vi "连接机柜.vi"(8 "error in (no error)":errorcluster) -> (0 "error out":errorcluster)   [LabVIEW 2015]
uses:
  Global/SeverGlobal.vi
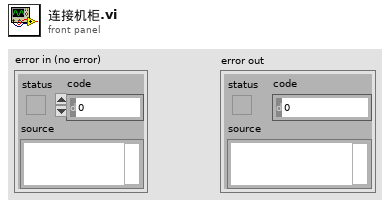
[diagram p1: front panel]
types:
  T1 = cluster{"IP_A":string, "PORT_A":i32, "IP_B":string, "PORT_B":i32, "IP_CLK":string, "PORT_CLK":i32, "IP_SWITCH":string, "PORT_SWITCH":i32}
  T2 = enum16{"Standard", "Buffered", "CRLF", "Immediate"}
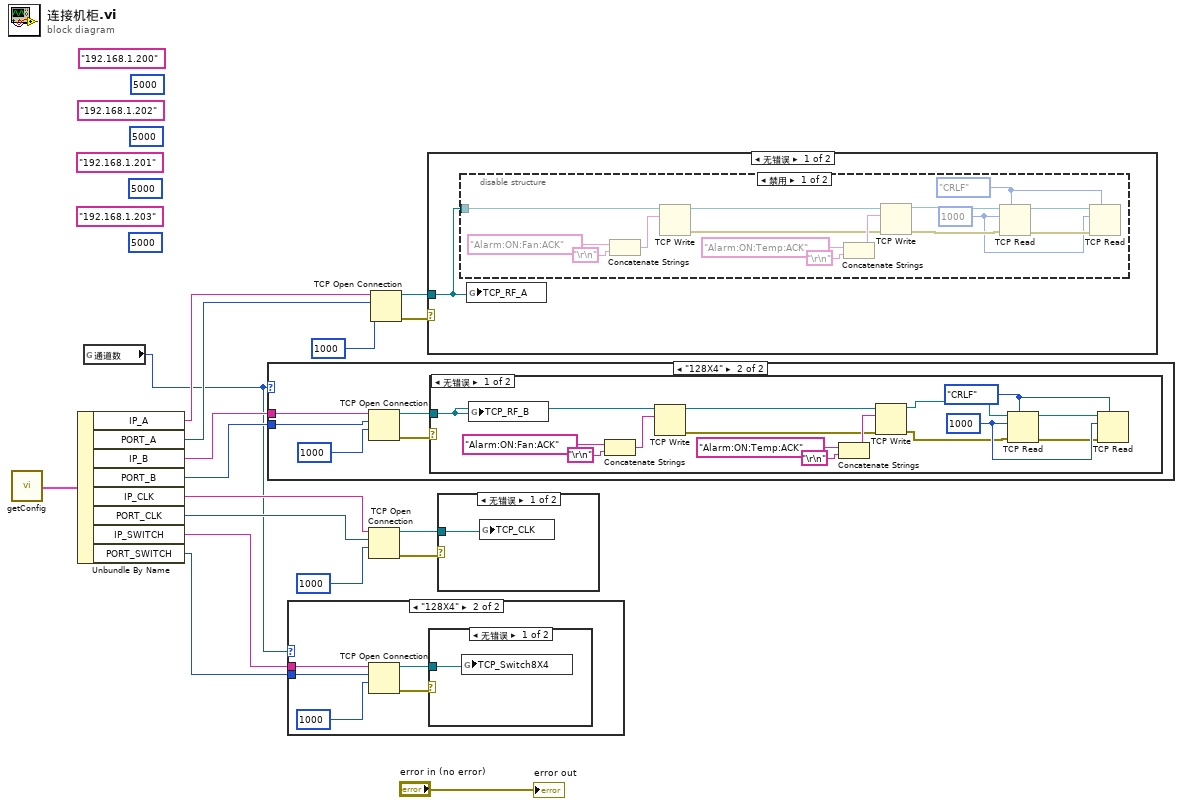
[diagram p0: block diagram]
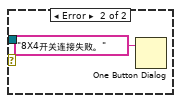
[diagram p3: hidden frame]
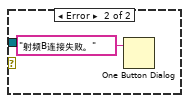
[diagram p5: hidden frame]
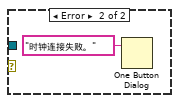
[diagram p6: hidden frame]
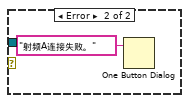
[diagram p8: hidden frame]
diagram:
  (unwired) u16 5000 ("PORT(RF)")
  (unwired) "192.168.1.203" ("IP(RF2)")
  (unwired) u16 5000 ("PORT(RF)")
  (unwired) "192.168.1.201" ("IP(RF2)")
  (unwired) u16 5000 ("PORT(RF)")
  (unwired) "192.168.1.202" ("IP(RF2)")
  (unwired) u16 5000 ("PORT(RF)")
  (unwired) "192.168.1.200" ("IP(RF2)")
  n1 = call "getConfig.vi"() -> ("config"=w10:T1)  [unwired: 1 in]
  n2 = Unbundle By Name(w10) -> ("IP_A"=w9:string, "PORT_A"=w8:i32, "IP_B"=w7:string, "PORT_B"=w6:i32, "IP_CLK"=w5:string, "PORT_CLK"=w4:i32, "IP_SWITCH"=w3:string, "PORT_SWITCH"=w2:i32)
  n3 = global read "SeverGlobal.vi" "通道数"() -> (w1:enum16{"64X4", "128X4"})
  n4 = case shown="\"128X4\"" w1 {
    tunnel: w7 -> [_ w19]
    tunnel: w6 -> [_ w18]
    frame "64X4", Default {
    }
    frame "128X4" {
      n5 = TCP Open Connection(address=w19, remote port or service name=w18, timeout ms (60000)=1000) -> (connection ID=w22:refnum<k5>, error out=w21:errorcluster)  [unwired: 2 in]
      n6 = case shown="无错误" w21 {
        tunnel: w22 -> [w37 _]
        frame No Error {
          w29 = 1000 ("bytes to read")
          w28 = T2."CRLF" ("mode (standard)")
          n7 = global write "SeverGlobal.vi" "TCP_RF_B"(w37) -> ()
          n8 = Concatenate Strings("Alarm:ON:Fan:ACK", "\r\n") -> (w34:string)
          n9 = TCP Write(connection ID=w37, data in=w34) -> (connection ID out=w33:refnum<k5>, error out=w23:errorcluster)  [unwired: 2 in, 1 out]
          n10 = Concatenate Strings("Alarm:ON:Temp:ACK", "\r\n") -> (w30:string)
          n11 = TCP Write(connection ID=w33, data in=w30, error in (no error)=w23) -> (connection ID out=w25:refnum<k5>, error out=w24:errorcluster)  [unwired: 1 in, 1 out]
          n12 = TCP Read(connection ID=w25, bytes to read=w29, error in (no error)=w24, 7:w28) -> (connection ID out=w26:refnum<k5>, error out=w27:errorcluster)  [unwired: 1 in, 1 out]
          n13 = TCP Read(connection ID=w26, bytes to read=w29, error in (no error)=w27, 7:w28) -> ()  [unwired: 1 in, 3 out]
        }
        frame Error {
          n14 = One Button Dialog(message="射频B连接失败。") -> ()  [unwired: 1 in, 1 out]
        }
      }
    }
  }
  n15 = case shown="\"128X4\"" w1 {
    tunnel: w3 -> [_ w40]
    tunnel: w2 -> [_ w39]
    frame "64X4", Default {
    }
    frame "128X4" {
      n16 = TCP Open Connection(address=w40, remote port or service name=w39, timeout ms (60000)=1000) -> (connection ID=w43:refnum<k5>, error out=w42:errorcluster)  [unwired: 2 in]
      n17 = case shown="无错误" w42 {
        tunnel: w43 -> [w44 _]
        frame No Error {
          n18 = global write "SeverGlobal.vi" "TCP_Switch8X4"(w44) -> ()
        }
        frame Error {
          n19 = One Button Dialog(message="8X4开关连接失败。") -> ()  [unwired: 1 in, 1 out]
        }
      }
    }
  }
  n20 = TCP Open Connection(address=w5, remote port or service name=w4, timeout ms (60000)=1000) -> (connection ID=w14:refnum<k5>, error out=w15:errorcluster)  [unwired: 2 in]
  n21 = TCP Open Connection(address=w9, remote port or service name=w8, timeout ms (60000)=1000) -> (connection ID=w16:refnum<k5>, error out=w17:errorcluster)  [unwired: 2 in]
  n22 = case shown="无错误" w17 {
    tunnel: w16 -> [w46 _]
    frame No Error {
      n23 = disable-structure shown="禁用" {
        disable-tunnel: w46 -> [w61 _]
        frame Disabled {
          w47 = 1000 ("bytes to read")
          w48 = T2."CRLF" ("mode (standard)")
          n24 = Concatenate Strings("Alarm:ON:Fan:ACK", "\r\n") -> (w58:string)
          n25 = TCP Write(connection ID=w61, data in=w58) -> (connection ID out=w57:refnum<k5>, error out=w49:errorcluster)  [unwired: 2 in, 1 out]
          n26 = Concatenate Strings("Alarm:ON:Temp:ACK", "\r\n") -> (w54:string)
          n27 = TCP Write(connection ID=w57, data in=w54, error in (no error)=w49) -> (connection ID out=w53:refnum<k5>, error out=w50:errorcluster)  [unwired: 1 in, 1 out]
          n28 = TCP Read(connection ID=w53, bytes to read=w47, error in (no error)=w50, 7:w48) -> (connection ID out=w52:refnum<k5>, error out=w51:errorcluster)  [unwired: 1 in, 1 out]
          n29 = TCP Read(connection ID=w52, bytes to read=w47, error in (no error)=w51, 7:w48) -> ()  [unwired: 1 in, 3 out]
        }
        frame Enabled {
        }
      }
      n30 = global write "SeverGlobal.vi" "TCP_RF_A"(w46) -> ()
    }
    frame Error {
      n31 = One Button Dialog(message="射频A连接失败。") -> ()  [unwired: 1 in, 1 out]
    }
  }
  n32 = case shown="无错误" w15 {
    tunnel: w14 -> [w63 _]
    frame No Error {
      n33 = global write "SeverGlobal.vi" "TCP_CLK"(w63) -> ()
    }
    frame Error {
      n34 = One Button Dialog(message="时钟连接失败。") -> ()  [unwired: 1 in, 1 out]
    }
  }
  "error out" <- "error in (no error)"
